vi "GetChild.vi"(8 "Error In":errorcluster, 10 "I":i32, 11 "reference in":refnum<class "Menu.lvclass">) -> (0 "Error Out":errorcluster, 2 "Return(LabVIEW Class)":refnum<class "MenuComponent.lvclass">, 3 "reference in":refnum<class "Menu.lvclass">)   [LabVIEW 2020, in "Menu.lvclass"]
uses:
  Menu.lvclass
  MenuComponent_class/MenuComponent.lvclass
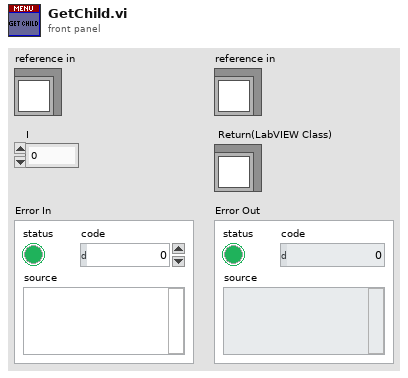
[diagram p1: front panel]
types:
  T1 = typedef "Menu.lvclass/ObjectAttributes.ctl" = cluster{"Items":refnum<class "MenuComponent.lvclass">[], "Name":string, "Description":string}
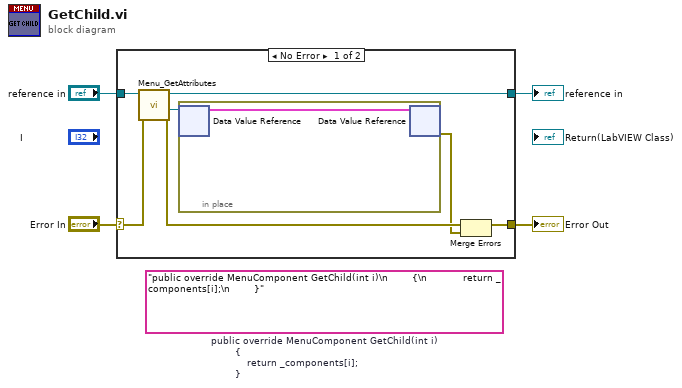
[diagram p0: block diagram]
diagram:
  (unwired) "public override MenuComponent GetChild(int i)\n        {\n            return _components[i];\n        }"  # public override MenuComponent GetChild(int i)         {             return _components[i];         }
  n1 = case shown="No Error" "Error In" {
    selector: "Error In" -> [w10 w14]
    tunnel: [w9 w14] -> w3
    tunnel: [w8 w13] -> w1
    tunnel: "reference in" -> [w11 w13]
    frame No Error {
      n2 = call "Menu_GetAttributes.vi"("error in (no error)"=w10, "reference in"=w11) -> ("error out"=w6:errorcluster, "DataRef"=w7:refnum<data-value>, "reference out"=w8:refnum<class "Menu.lvclass">)  [unwired: 6 in, 1 out]
      n3 = in-place {
        n4 = in-place-dvr #1(w7) -> (w12:T1)  [unwired: 1 out]
        n5 = in-place-dvr #1(w12) -> (w5:errorcluster)  [unwired: 1 out]
      }
      n6 = Merge Errors(w6, w5) -> (w9:errorcluster)
    }
    frame Error {
    }
  }
  "Error Out" <- w3
  "reference in" <- w1
